vi "exit.vi"(8 "error in (no error)":errorcluster, 11 "Input":string) -> (0 "error out":errorcluster, 3 "Output":string)   [LabVIEW 2014]
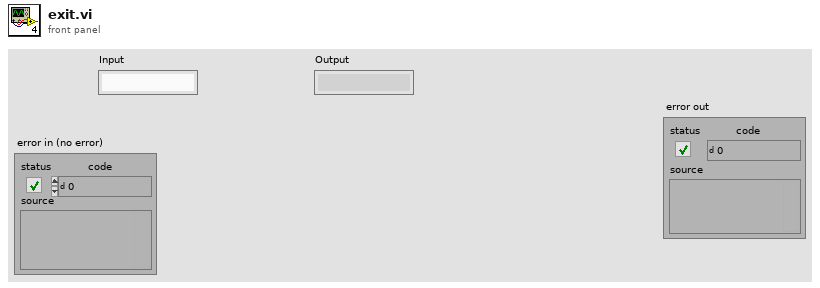
[diagram p1: front panel]
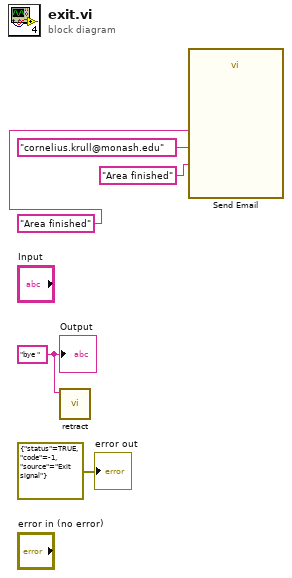
[diagram p0: block diagram]
diagram:
  w4 = "bye " ("string")
  n1 = call "retract.vi"("Input"=w4) -> ()  [unwired: 9 in, 2 out]
  n2 = call "Send Email"("Message"="Area finished" ("Subject"), "Subject"="Area finished", "Recipients"="cornelius.krull@monash.edu") -> ()  [unwired: 8 in, 1 out]
  "Output" <- w4
  "error out" <- errorcluster {"status"=TRUE, "code"=-1, "source"="Exit signal"} ("error out")
